vi "dummy_data_sendout.vi"() -> ()   [LabVIEW 2014]
uses:
  Common/LaserScan.ctl
  Common/Odometry.ctl
  Common/TwistCovariance.ctl
  <userlib>/ROS for LabVIEW Software/ROS/Code/Console/Servers/ServerSubs/TopicDef.ctl
  <userlib>/ROS for LabVIEW Software/ROS/Code/SubVIs/_ROSDirection.ctl
  <userlib>/ROS for LabVIEW Software/ROS/Code/_ROSDefinition.vi
panel:
  in  "laser_frame_id":string="base_laser"
  in  "stop":bool
  in  "odometry_frame":string="odometry"
  in  "Y Velocity (m/s)":dbl(slide) min=-1.0 max=1.0 scale=-0.3..0.3
  in  "X Velocity (m/s)":dbl(slide) min=-1.0 max=1.0 scale=-0.3..0.3
  in  "Angular Velocity (rad/s)":dbl(slide) min=-2.0 max=2.0 scale=2.0..-2.0
  out "Y Velocity Feedback":dbl(slide) scale=-0.3..0.3
  out "X Velocity Feedback":dbl(slide) scale=-0.3..0.3
  out "Angular Velocity Feedback":dbl(slide) scale=2.0..-2.0
  out "end":bool
  out "OmniDynamics out":T1
  out "LaserScan":T3
  in  "ROS Master":string="172.16.0.10:11311"
  in  "base_link":string="base_link"
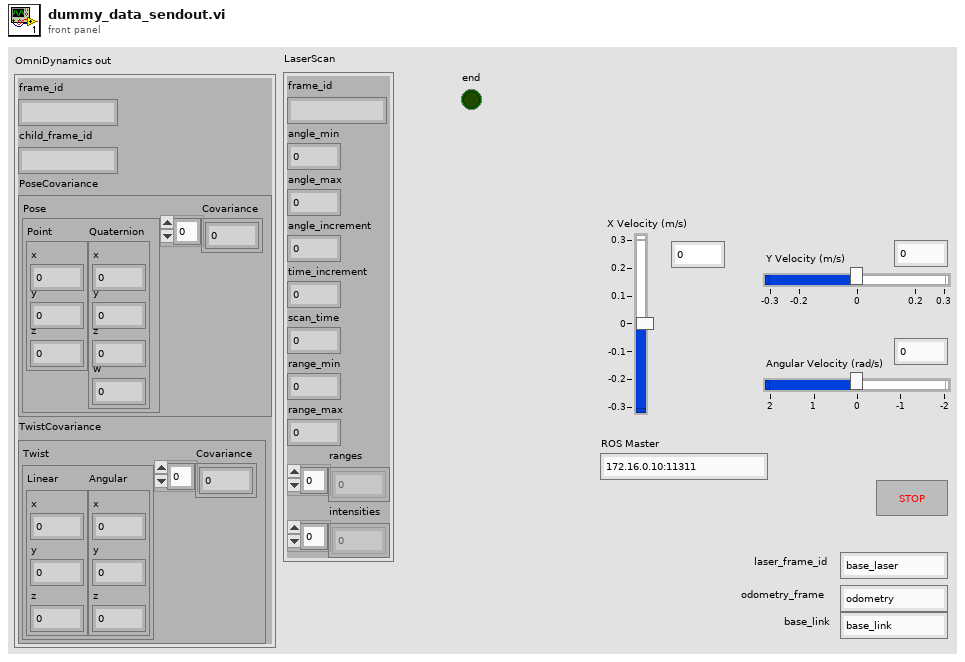
[diagram p1: front panel]
types:
  T1 = typedef "Odometry.ctl" = cluster{"frame_id":string, "child_frame_id":string, "PoseCovariance":cluster{"Pose":cluster{"Point":cluster{"x":dbl, "y":dbl, "z":dbl}, "Quaternion":cluster{"x":dbl, "y":dbl, "z":dbl, "w":dbl}}, "Covariance":dbl[]}, "TwistCovariance":T2}
  T2 = typedef "TwistCovariance.ctl" = cluster{"Twist":cluster{"Linear":cluster{"x":dbl, "y":dbl, "z":dbl}, "Angular":cluster{"x":dbl, "y":dbl, "z":dbl}}, "Covariance":dbl[]}
  T3 = typedef "LaserScan.ctl" = cluster{"frame_id":string, "angle_min":dbl, "angle_max":dbl, "angle_increment":dbl, "time_increment":dbl, "scan_time":dbl, "range_min":dbl, "range_max":dbl, "ranges":dbl[], "intensities":dbl[]}
  T4 = typedef "TopicDef.ctl" = cluster{"Topic":string, "Type":string, "Action":T5, "Update (ms)":u16, "queue size":u16}
  T5 = typedef "_ROSDirection.ctl" = enum16{"Node", "Publisher", "Subscriber", "ServiceClient", "ServiceProvider"}
  T6 = typedef "_ROSControl.ctl" = cluster{"topic port":u16, "Node":string, "topic":string, "type":string, "node port":u16, "error ":errorcluster, "Direction":T5, "Update (ms)":u16, "FIFO size":u16}
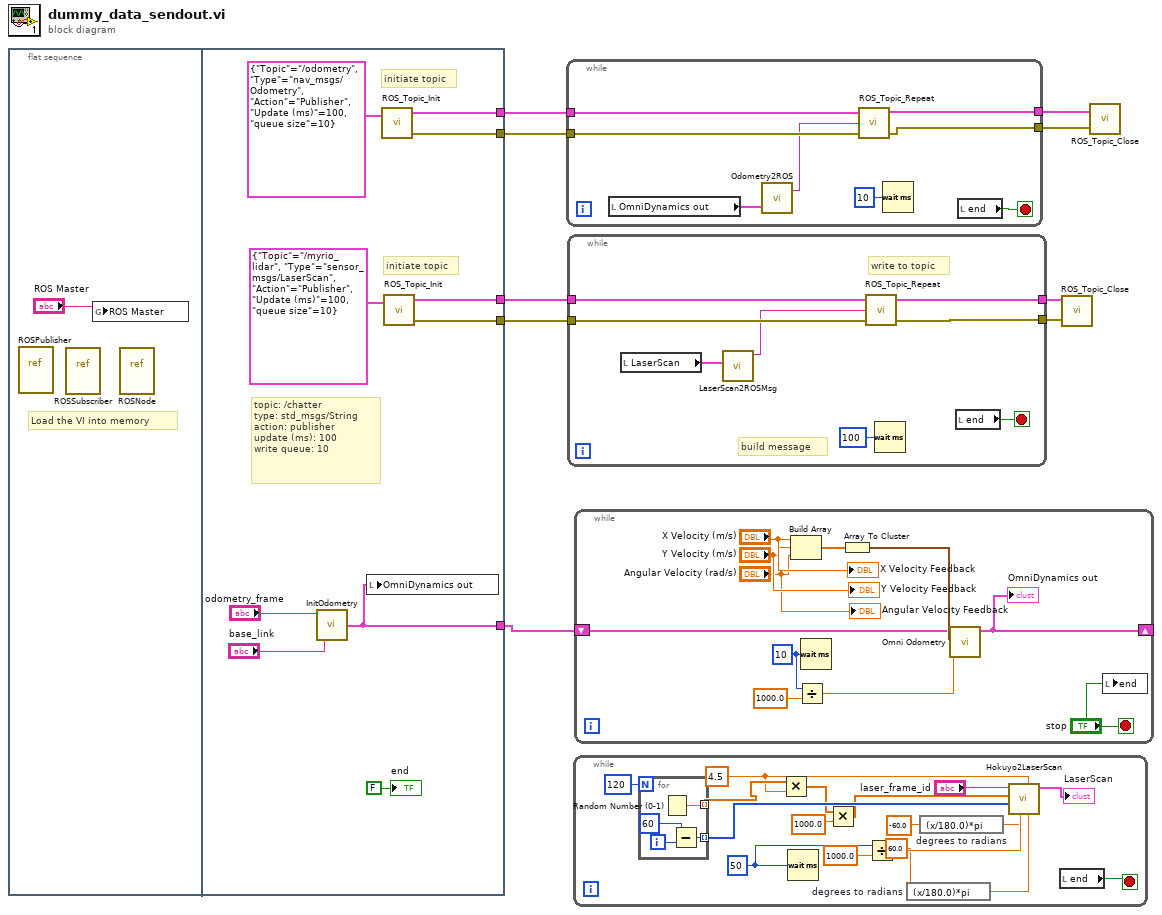
[diagram p0: block diagram]
diagram:
  n1 = flat-sequence {
    tunnel: [w19] -> w9
    tunnel: [w18] -> w8
    tunnel: [w17] -> w5
    tunnel: [w16] -> w4
    tunnel: [w12] -> w1
    frame #0 {
      # "Load the VI into memory"
      n2 = vi-ref <userlib>:"ROSPublisher.vi"() -> ()  [unwired: 1 out]
      n3 = vi-ref <userlib>:"ROSSubscriber.vi"() -> ()  [unwired: 1 out]
      n4 = global write "_ROSDefinition.vi" "ROS Master"("ROS Master") -> ()
      n5 = vi-ref <userlib>:"ROSNode.vi"() -> ()  [unwired: 1 out]
    }
    frame #1 {
      # "initiate topic"
      # "topic: /chatter\ntype: std_msgs/String\naction: publisher\nupdate (ms): 100\nwrite queue: 10"
      # "initiate topic"
      n6 = call "InitOdometry.vi"("child_frame_id"="base_link", "frame_id"="odometry_frame") -> ("OmniDynamics out"=w12:T1)
      n7 = local write "OmniDynamics out"(w12) -> ()
      n8 = call <userlib>:"ROS_Topic_Init.vi"("Definitions"=T4 {"Topic"="/odometry", "Type"="nav_msgs/Odometry", "Action"=enum."Publisher", "Update (ms)"=100, "queue size"=10}) -> ("ROS out"=w17:T6, "error out"=w16:errorcluster)  [unwired: 2 in]
      n9 = call <userlib>:"ROS_Topic_Init.vi"("Definitions"=T4 {"Topic"="/myrio_lidar", "Type"="sensor_msgs/LaserScan", "Action"=enum."Publisher", "Update (ms)"=100, "queue size"=10}) -> ("ROS out"=w19:T6, "error out"=w18:errorcluster)  [unwired: 2 in]
      "end" <- FALSE ("end")
    }
  }
  n10 = while {
    tunnel: w5 -> [w26]
    tunnel: w4 -> [w25]
    tunnel: [w24] -> w3
    tunnel: [w23] -> w2
    stop <- w28 stop-if-true
    n11 = local read "OmniDynamics out"() -> (w22:T1)
    n12 = call "Odometry2ROS.vi"("OmniDynamics out"=w22) -> ("msg out"=w21:string)  [unwired: 2 in]
    n13 = call <userlib>:"ROS_Topic_Repeat.vi"("error in (no error)"=w25, "Msg in"=w21, "ROS in"=w26) -> ("error out"=w23:errorcluster, "ROS out"=w24:T6)  [unwired: 1 in]
    n14 = Wait (ms)(milliseconds to wait=u32 10) -> ()  [unwired: 1 out]
    n15 = local read "end"() -> (w28:bool)
  }
  n16 = while {
    tunnel: w9 -> [w36]
    tunnel: w8 -> [w35]
    tunnel: [w34] -> w7
    tunnel: [w33] -> w6
    stop <- w32 stop-if-true
    # "build message"
    # "write to topic"
    n17 = local read "LaserScan"() -> (w31:T3)
    n18 = call "LaserScan2ROSMsg.vi"("LaserScan"=w31) -> ("msg out"=w30:string)  [unwired: 10 in]
    n19 = call <userlib>:"ROS_Topic_Repeat.vi"("error in (no error)"=w35, "Msg in"=w30, "ROS in"=w36) -> ("error out"=w33:errorcluster, "ROS out"=w34:T6)  [unwired: 1 in]
    n20 = Wait (ms)(milliseconds to wait=u32 100) -> ()  [unwired: 1 out]
    n21 = local read "end"() -> (w32:bool)
  }
  n22 = while {
    stop <- w53 stop-if-true
    w45 = 4.5 ("range_max")
    w48 = u32 50 ("milliseconds to wait")
    n23 = for {
      N: 120 -> [_]
      tunnel: [w57] -> w46 mode=indexing
      tunnel: [w54] -> w50 mode=indexing
      i -> [w56]
      n24 = Random Number (0-1)() -> (number: 0 to 1=w57:dbl)
      n25 = Subtract(x=w56, y=60) -> (x-y=w54:i32)
    }
    n26 = Multiply(x=w46, y=w45) -> (x*y=w43:dbl[])
    n27 = Wait (ms)(milliseconds to wait=w48) -> ()  [unwired: 1 out]
    n28 = Multiply(x=w43, y=1000.0) -> (x*y=w41:dbl[])
    n29 = Divide(x=w48, y=1000.0) -> (x/y=w47:dbl)
    n30 = expression code="(x/180.0)*pi" "degrees to radians"(60.0 ("angle_max")) -> (w37:dbl)
    n31 = expression code="(x/180.0)*pi" "degrees to radians"(-60.0 ("angle_min")) -> (w40:dbl)
    n32 = call "Hokuyo2LaserScan.vi"("angle_max"=w37, "range_max"=w45, "angle_min"=w40, "scan_time"=w47, "Direction"=w50, "Magnitude"=w41, "frame_id"="laser_frame_id") -> ("LaserScan"=→"LaserScan":T3)  [unwired: 4 in]
    n33 = local read "end"() -> (w53:bool)
  }
  n34 = while {
    shift-right: [w62] -> _
    shift-left: w1 -> [w63]
    stop <- "stop" stop-if-true
    w68 = u32 10 ("milliseconds to wait")
    n35 = Build Array("X Velocity (m/s)", "Y Velocity (m/s)", "Angular Velocity (rad/s)") -> (w65:dbl[])
    n36 = Divide(x=w68, y=1000.0) -> (x/y=w66:dbl)
    n37 = Wait (ms)(milliseconds to wait=w68) -> ()  [unwired: 1 out]
    n38 = Array To Cluster(array=w65) -> (cluster=w64:cluster{"[0]":dbl, "[1]":dbl, "[2]":dbl})
    n39 = call "Omni Odometry.vi"("dt"=w66, "TaimiOmniVelocity"=w64, "OmniDynamics in"=w63) -> ("OmniDynamics out"=w62:T1)  [unwired: 8 in]
    "OmniDynamics out" <- w62
    n40 = local write "end"("stop") -> ()
    "X Velocity Feedback" <- "X Velocity (m/s)"
    "Y Velocity Feedback" <- "Y Velocity (m/s)"
    "Angular Velocity Feedback" <- "Angular Velocity (rad/s)"
  }
  n41 = call <userlib>:"ROS_Topic_Close.vi"("error in"=w6, "ROS in"=w7) -> ()  [unwired: 2 in, 1 out]
  n42 = call <userlib>:"ROS_Topic_Close.vi"("error in"=w2, "ROS in"=w3) -> ()  [unwired: 2 in, 1 out]
